vi "Chrg_Dschrg_new.vi"(0 "Data Task in":refnum<k21>, 1 "data task error in":errorcluster, 2 "#DAQ outputs (1-13)":i32, 3 "PS type":enum16{"NHR", "ITECH"}(ring), 4 "PS VISA in":refnum<visa-resource-name>, 5 "PS error in":errorcluster caption="NHR error in (no error)", 6 "DischargeCyclePath":path=path "C:/Users/ga11/Desktop/VI/results/3PtestCharge.lvm" caption="Filename", 7 "Battery Type":enum16{"30Q", "40T"}(ring), 8 "Charge/discharge":enum8{"Charge", "Discharge"}(ring), 9 "Charge/Discharge Voltage Setpoint":dbl format="%#.6g", 10 "CC or CCCV":enum16{"CC", "CCCV"}(ring), 11 "Current Setpoint":dbl format="%#.6g", 12 "Output Safety":T1, 13 "Current Cutoff":dbl) -> (14 "data task out":refnum<k21>, 15 "data task error out":errorcluster, 18 "PS VIS resource name out":refnum<visa-resource-name>, 19 "PS error out":errorcluster)   [LabVIEW 2020]
uses:
  Drivers-Essentials/NH Research Regenerative Test Series.lvlib
  Drivers-IT-M3400/IT-M3400.lvlib
  Drivers-Essentials/Read (Ave Current).vi
  Drivers-NHR-9200/NHR/Public/Data/Low Level/Fetch (Ave Voltage).vi
  <instrlib>/NH Research Regenerative Test Series/Public/Configure/Output Safety.ctl
panel:
  out "Read Ave Current (A)":dbl
  out "Read Ave Voltage (V)":dbl
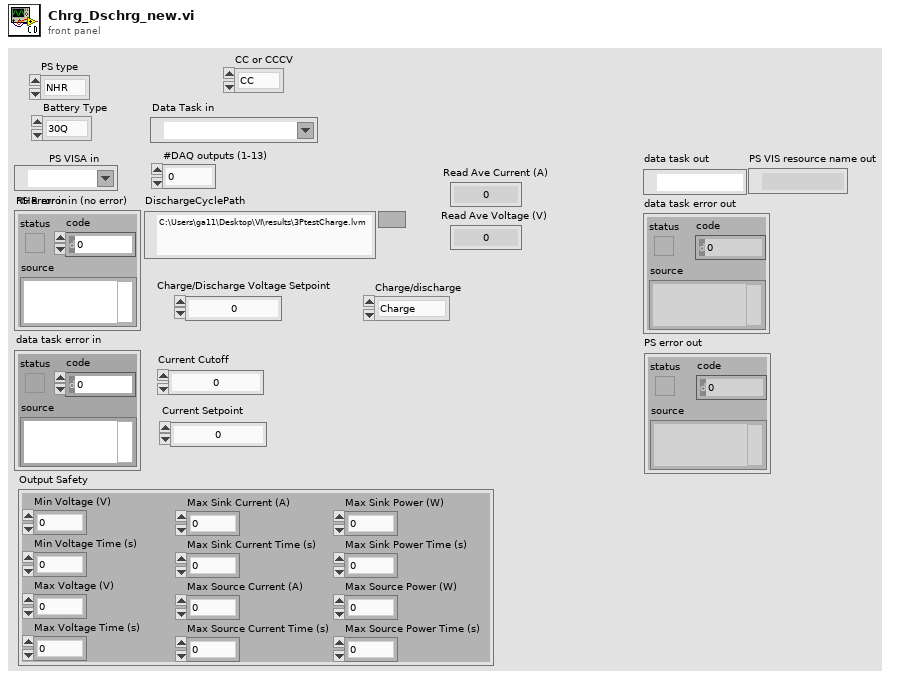
[diagram p1: front panel]
types:
  T1 = typedef "NH Research Regenerative Test Series.lvlib/Output Safety.ctl" = cluster{"Min Voltage (V)":dbl, "Min Voltage Time (s)":dbl, "Max Voltage (V)":dbl, "Max Voltage Time (s)":dbl, "Max Sink Current (A)":dbl, "Max Sink Current Time (s)":dbl, "Max Source Current (A)":dbl, "Max Source Current Time (s)":dbl, "Max Sink Power (W)":dbl, "Max Sink Power Time (s)":dbl, "Max Source Power (W)":dbl, "Max Source Power Time (s)":dbl}
  T2 = cluster{"Voltage Enabled":bool, "Current Enabled":bool, "Power Enabled":bool, "Resistance Enabled":bool}
  T3 = cluster{"Baud Rate":u32, "Parity":u16, "Data Bits":u16, "Stop Bits":u16, "Flow Control":u16}
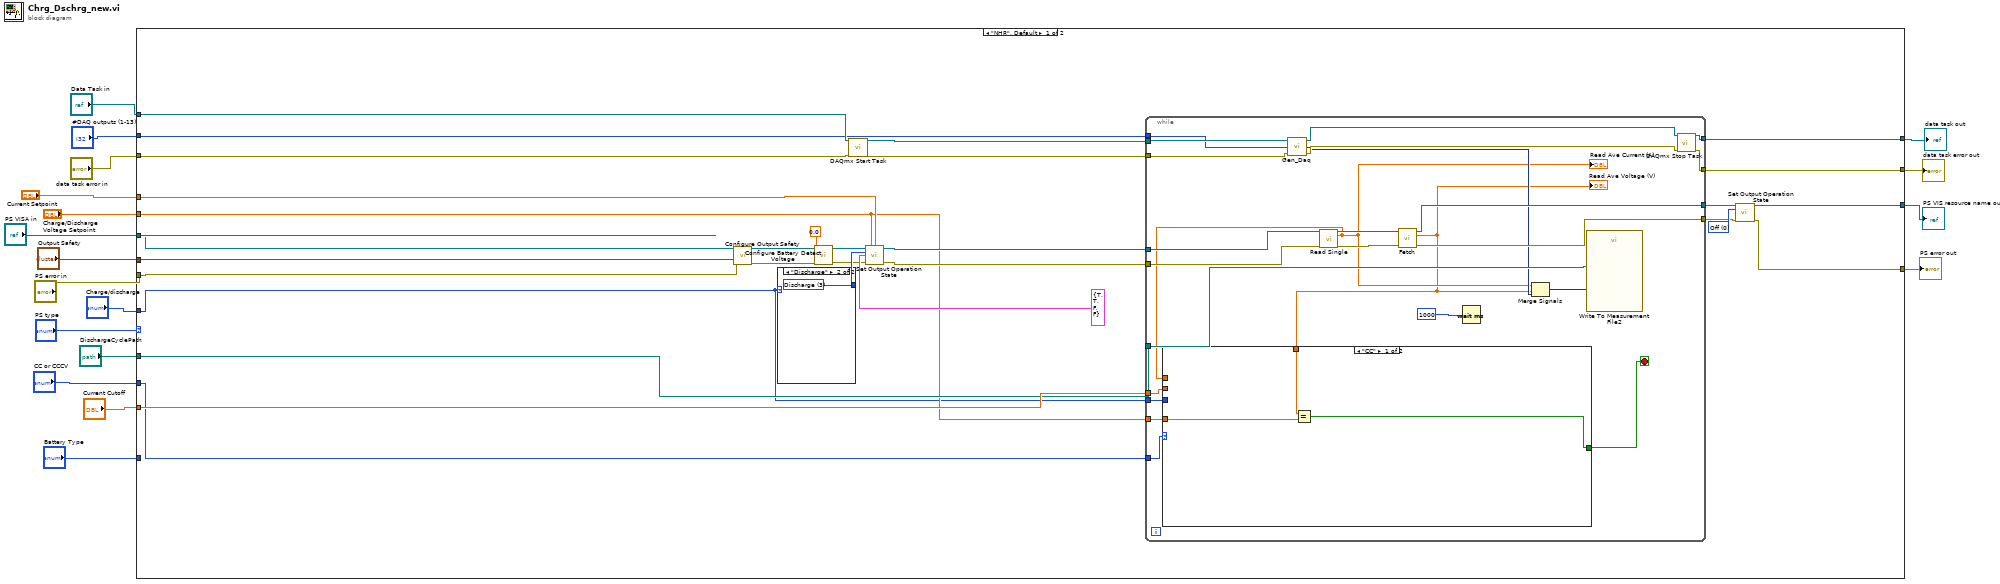
[diagram p0: block diagram]
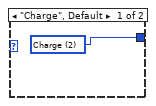
[diagram p2: hidden frame]
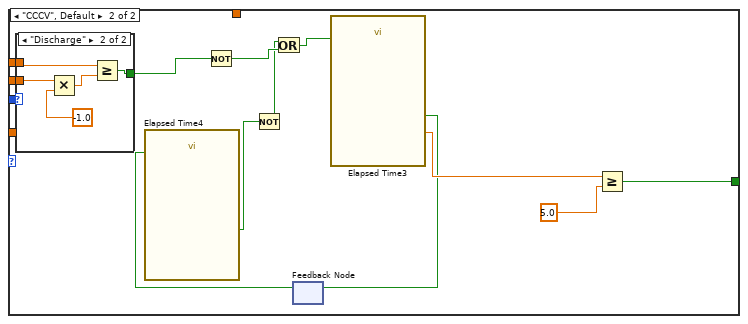
[diagram p3: hidden frame]
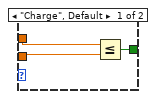
[diagram p4: hidden frame]
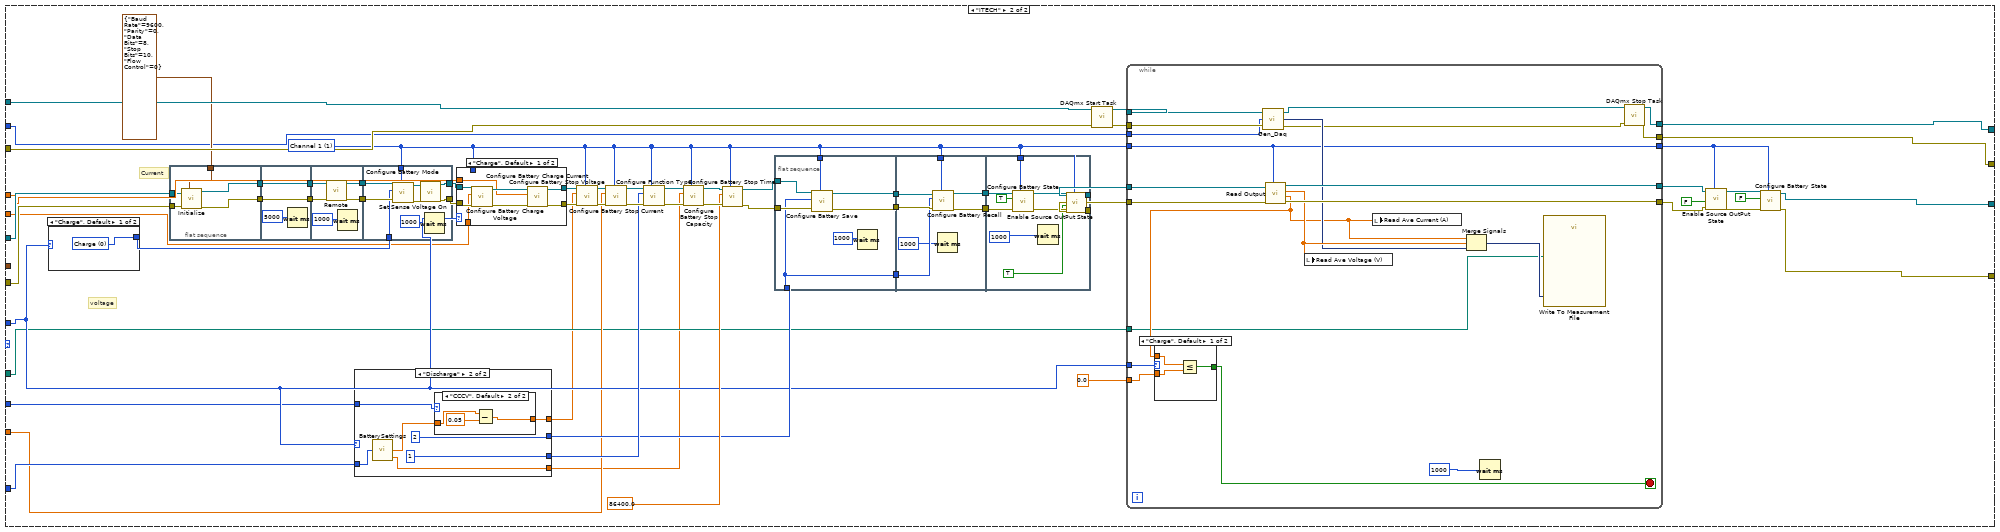
[diagram p5: hidden frame]
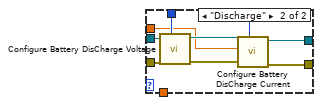
[diagram p6: hidden frame]
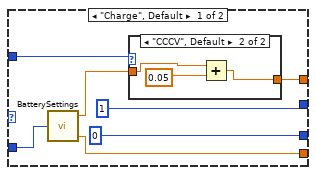
[diagram p7: hidden frame]
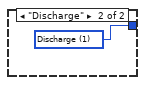
[diagram p10: hidden frame]
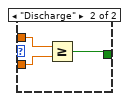
[diagram p11: hidden frame]
diagram:
  n1 = case shown="\"NHR\", Default" "PS type" {
    tunnel: "Charge/Discharge Voltage Setpoint" -> [w25 w104]
    tunnel: "Current Setpoint" -> [w27 w105]
    tunnel: "Current Cutoff" -> [w46 w109]
    tunnel: "DischargeCyclePath" -> [w43 w108]
    tunnel: "Data Task in" -> [w40 w150]
    tunnel: "data task error in" -> [w39 w151]
    tunnel: "PS VISA in" -> [w20 w107]
    tunnel: "PS error in" -> [w21 w106]
    tunnel: [w34 w149] -> w10
    tunnel: [w33 w147] -> w9
    tunnel: [w32 w148] -> w8
    tunnel: [w31 w146] -> w7
    tunnel: "#DAQ outputs (1-13)" -> [w28 w113]
    tunnel: "Battery Type" -> [_ w110]
    tunnel: "Charge/discharge" -> [w24 w111]
    tunnel: "CC or CCCV" -> [w26 w103]
    tunnel: "Output Safety" -> [w19 _]
    frame "NHR", Default {
      w38 = 0 items=["Off", "Standby", "Charge", "Discharge", "Battery"] ("Mode (0: Off)")
      n2 = call <instrlib>:"Configure Output Safety.vi"("VISA resource name"=w20, "Output Safety"=w19, "error in (no error)"=w21) -> ("VISA resource name out"=w23:refnum<visa-resource-name>, "error out"=w22:errorcluster)  [unwired: 11 in]
      n3 = case shown="\"Discharge\"" w24 {
        tunnel: [w49 w50] -> w44
        frame "Charge", Default {
          w49 = 2 items=["Off", "Standby", "Charge", "Discharge", "Battery"] ("Mode (0: Off)")
        }
        frame "Discharge" {
          w50 = 3 items=["Off", "Standby", "Charge", "Discharge", "Battery"] ("Mode (0: Off)")
        }
      }
      n4 = call "Configure Battery Detect Voltage.vi"("VISA resource name"=w23, "Battery Detect Voltage (0V)"=0.0, "error in (no error)"=w22) -> ("VISA resource name out"=w37:refnum<visa-resource-name>, "error out"=w36:errorcluster)  [unwired: 11 in]
      n5 = call <vilib>:"DAQmx Start Task.vi"("task/channels in"=w40, "error in"=w39) -> ("task out"=w42:refnum<k21>, "error out"=w41:errorcluster)  [unwired: 12 in]
      n6 = call "Set Output Operation State.vi"("VISA resource name"=w37, "Voltage Setpoint (0 V)"=w25, "Current Setpoint (0 A)"=w27, "Mode (0: Off)"=w44, "Enable"=T2 {"Voltage Enabled"=TRUE, "Current Enabled"=TRUE, "Power Enabled"=FALSE, "Resistance Enabled"=FALSE}, "error in (no error)"=w36) -> ("VISA resource name out"=w48:refnum<visa-resource-name>, "error out"=w47:errorcluster)  [unwired: 8 in]
      n7 = while {
        tunnel: w48 -> [w72]
        tunnel: w47 -> [w71]
        tunnel: w46 -> [w56]
        tunnel: w41 -> [w61]
        tunnel: w42 -> [w62]
        tunnel: w43 -> [w67]
        tunnel: [w66] -> w34
        tunnel: [w65] -> w32
        tunnel: [w64] -> w30
        tunnel: [w63] -> w29
        tunnel: w28 -> [w60]
        tunnel: w26 -> [w54]
        tunnel: w25 -> [w52]
        tunnel: w24 -> [w51]
        stop <- w68 stop-if-true
        n8 = call "Gen_Daq.vi"("error in"=w61, "#DAQ outputs (1-13)"=w60, "task/channels in"=w62) -> ("error out"=w58:errorcluster, "DaQ_output"=w57:dynamicdata, "task out"=w59:refnum<k21>)
        n9 = call-poly "Read Single.vi"("VISA resource name"=w72, "error in (no error)"=w71) -> ("VISA resource name out"=w73:refnum<visa-resource-name>, "Ave Current (A)"=w55:dbl, "error out"=w74:errorcluster)  [unwired: 11 in]
        "Read Ave Current (A)" <- w55
        n10 = call-poly "Fetch.vi"("VISA resource name"=w73, "error in (no error)"=w74) -> ("VISA resource name out"=w64:refnum<visa-resource-name>, "Ave Voltage (V)"=w53:dbl, "error out"=w63:errorcluster)  [unwired: 11 in]
        "Read Ave Voltage (V)" <- w53
        n11 = case shown="\"CC\"" w54 {
          tunnel: [w75 w84] -> w68
          tunnel: w56 -> [_ w81]
          tunnel: w55 -> [_ w80]
          tunnel: w53 -> [w77 _]
          tunnel: w52 -> [w76 _]
          tunnel: w51 -> [_ w78]
          frame "CC" {
            n12 = Equal?(x=w77, y=w76) -> (x = y?=w75:bool)
          }
          frame "CCCV", Default {
            n13 = case shown="\"Discharge\"" w78 {
              tunnel: w81 -> [w92 w97]
              tunnel: w80 -> [w93 w95]
              tunnel: [w91 w94] -> w79
              frame "Charge", Default {
                n14 = Less Or Equal?(x=w93, y=w92) -> (x <= y?=w91:bool)
              }
              frame "Discharge" {
                n15 = Multiply(x=w97, y=-1.0) -> (x*y=w96:dbl)
                n16 = Greater Or Equal?(x=w95, y=w96) -> (x >= y?=w94:bool)
              }
            }
            n17 = Not(x=w79) -> (.not. x?=w90:bool)
            n18 = feedback #1() -> (w82:bool)  [unwired: 1 in]
            n19 = call "Elapsed Time4"("Reset"=w82) -> ("Time has Elapsed"=w89:bool)  [unwired: 11 in, 7 out]
            n20 = Not(x=w89) -> (.not. x?=w88:bool)
            n21 = Or(x=w88, y=w90) -> (x .or. y?=w87:bool)
            n22 = call "Elapsed Time3"("Reset"=w87) -> ("Elapsed Time (s)"=w86:dbl, "Time has Elapsed"=w83:bool)  [unwired: 11 in, 6 out]
            n23 = feedback-in #1(w83) -> ()
            n24 = Greater Or Equal?(x=w86, y=5.0) -> (x >= y?=w84:bool)
          }
        }
        n25 = Wait (ms)(milliseconds to wait=1000) -> ()  [unwired: 1 out]
        n26 = Merge Signals "Merge Signals"(w55, w53, w57) -> (w70:dynamicdata)
        n27 = call "Write To Measurement File2"("Signals"=w70, "Filename"=w67) -> ()  [unwired: 15 in, 3 out]
        n28 = call <vilib>:"DAQmx Stop Task.vi"("task/channels in"=w59, "error in"=w58) -> ("task out"=w66:refnum<k21>, "error out"=w65:errorcluster)  [unwired: 12 in]
      }
      n29 = call "Set Output Operation State.vi"("VISA resource name"=w30, "Mode (0: Off)"=w38, "error in (no error)"=w29) -> ("VISA resource name out"=w33:refnum<visa-resource-name>, "error out"=w31:errorcluster)  [unwired: 11 in]
    }
    frame "ITECH" {
      w114 = 1 items=["Channel 1"=1, "Channel 2"=2, "Channel 3"=3, "Channel 4"=4, "Channel 5"=5, "Channel 6"=6, "Channel 7"=7, "Channel 8"=8, "Channel 8"=9, "Channel 10"=10, "Channel 11"=11, "Channel 12"=12, "Channel 13"=13, "Channel 14"=14, "Channel 15"=15, "Channel 16"=16] ("Channel")
      # "voltage"
      # "Current"
      n30 = case shown="\"Charge\", Default" w111 {
        tunnel: [w244 w245] -> w124
        frame "Charge", Default {
          w244 = u8 0 items=["Charge", "Discharge"] ("Battery Mode")
        }
        frame "Discharge" {
          w245 = u8 1 items=["Charge", "Discharge"] ("Battery Mode")
        }
      }
      n31 = flat-sequence {
        tunnel: [w160] -> w139
        tunnel: [w161] -> w138
        tunnel: T3 {"Baud Rate"=9600, "Parity"=0, "Data Bits"=8, "Stop Bits"=10, "Flow Control"=0} ("Serial Configuration") -> [w164]
        tunnel: w106 -> [w163]
        tunnel: w107 -> [w162]
        tunnel: w139 -> [w167]
        tunnel: [w167] -> w137
        tunnel: w138 -> [w166]
        tunnel: [w166] -> w136
        tunnel: [w172] -> w135
        tunnel: [w171] -> w134
        tunnel: w137 -> [w170]
        tunnel: w136 -> [w169]
        tunnel: w135 -> [w178]
        tunnel: w134 -> [w180]
        tunnel: w114 -> [w181]
        tunnel: w124 -> [w179]
        tunnel: [w174] -> w100
        tunnel: [w173] -> w99
        frame #0 {
          n32 = call "Initialize.vi"("Serial Configuration"=w164, "error in"=w163, "VISA resource name"=w162) -> ("error out"=w161:errorcluster, "VISA resource name out"=w160:refnum<visa-resource-name>)  [unwired: 7 in]
        }
        frame #1 {
          n33 = Wait (ms)(milliseconds to wait=5000) -> ()  [unwired: 1 out]
        }
        frame #2 {
          n34 = call "Remote.vi"("error in"=w169, "VISA resource name"=w170) -> ("error out"=w171:errorcluster, "VISA resource name out"=w172:refnum<visa-resource-name>)  [unwired: 8 in]
          n35 = Wait (ms)(milliseconds to wait=1000) -> ()  [unwired: 1 out]
        }
        frame #3 {
          n36 = call "Configure Battery Mode.vi"("Channel"=w181, "error in"=w180, "Battery Mode"=w179, "VISA resource name"=w178) -> ("error out"=w175:errorcluster, "VISA resource name out"=w176:refnum<visa-resource-name>)  [unwired: 6 in]
          n37 = call "Set Sense Voltage On.vi"("error in"=w175, "VISA resource name"=w176) -> ("error out"=w174:errorcluster, "VISA resource name out"=w173:refnum<visa-resource-name>)  [unwired: 8 in]
          n38 = Wait (ms)(milliseconds to wait=1000) -> ()  [unwired: 1 out]
        }
      }
      n39 = case shown="\"Discharge\"" w111 {
        tunnel: w110 -> [w228 w233]
        tunnel: [u8 0 ("File") u8 1 ("File")] -> w118
        tunnel: [u8 1 ("File") u8 2 ("File")] -> w117
        tunnel: [w225 w237] -> w101
        tunnel: w103 -> [w222 w236]
        tunnel: [w223 w235] -> w102
        frame "Charge", Default {
          n40 = call "BatterySettings.vi"("Battery Type"=w228) -> ("RatedCapacity (Ah)"=w225:dbl, "Max Voltage (V)"=w224:dbl)  [unwired: 2 in, 1 out]
          n41 = case shown="\"CCCV\", Default" w222 {
            tunnel: w224 -> [w229 w231]
            tunnel: [w229 w230] -> w223
            frame "CC" {
            }
            frame "CCCV", Default {
              n42 = Add(x=w231, y=0.05) -> (x+y=w230:dbl)
            }
          }
        }
        frame "Discharge" {
          n43 = call "BatterySettings.vi"("Battery Type"=w233) -> ("RatedCapacity (Ah)"=w237:dbl, "Min Voltage (V)"=w234:dbl)  [unwired: 2 in, 1 out]
          n44 = case shown="\"CCCV\", Default" w236 {
            tunnel: w234 -> [w240 w242]
            tunnel: [w240 w241] -> w235
            frame "CC" {
            }
            frame "CCCV", Default {
              n45 = Subtract(x=w242, y=0.05) -> (x-y=w241:dbl)
            }
          }
        }
      }
      n46 = case shown="\"Charge\", Default" w111 {
        tunnel: w99 -> [w206 w221]
        tunnel: w100 -> [w213 w220]
        tunnel: [w209 w217] -> w129
        tunnel: [w208 w216] -> w128
        tunnel: w114 -> [_ w215]
        tunnel: w105 -> [w210 w214]
        tunnel: w104 -> [w207 _]
        frame "Charge", Default {
          n47 = call "Configure Battery Charge Voltage.vi"("error in"=w213, "Charge Voltage(V)"=w207, "VISA resource name"=w206) -> ("error out"=w211:errorcluster, "VISA resource name out"=w212:refnum<visa-resource-name>)  [unwired: 6 in]
          n48 = call "Configure Battery Charge Current.vi"("error in"=w211, "Charge Current(A)"=w210, "VISA resource name"=w212) -> ("error out"=w208:errorcluster, "VISA resource name out"=w209:refnum<visa-resource-name>)  [unwired: 7 in]
        }
        frame "Discharge" {
          n49 = call "Configure Battery DisCharge Voltage.vi"("Channel"=w215, "error in"=w220, "VISA resource name"=w221) -> ("error out"=w218:errorcluster, "VISA resource name out"=w219:refnum<visa-resource-name>)  [unwired: 7 in]
          n50 = call "Configure Battery DisCharge Current.vi"("Channel"=w215, "error in"=w218, "Discharge Current(A)"=w214, "VISA resource name"=w219) -> ("error out"=w216:errorcluster, "VISA resource name out"=w217:refnum<visa-resource-name>)  [unwired: 6 in]
        }
      }
      n51 = call "Configure Battery Stop Voltage.vi"("Channel"=w114, "error in"=w128, "Stop Voltage(V)"=w102, "VISA resource name"=w129) -> ("error out"=w132:errorcluster, "VISA resource name out"=w133:refnum<visa-resource-name>)  [unwired: 6 in]
      n52 = call "Configure Battery Stop Current.vi"("Channel"=w114, "error in"=w132, "Stop Current(A)"=w109, "VISA resource name"=w133) -> ("error out"=w120:errorcluster, "VISA resource name out"=w122:refnum<visa-resource-name>)  [unwired: 6 in]
      n53 = call "Configure Function Type.vi"("Channel"=w114, "error in"=w120, "Function Type"=w118, "VISA resource name"=w122) -> ("error out"=w119:errorcluster, "VISA resource name out"=w121:refnum<visa-resource-name>)  [unwired: 6 in]
      n54 = call "Configure Battery Stop Capacity.vi"("Channel"=w114, "error in"=w119, "Stop Capacity(Ah)"=w101, "VISA resource name"=w121) -> ("error out"=w130:errorcluster, "VISA resource name out"=w131:refnum<visa-resource-name>)  [unwired: 6 in]
      n55 = call "Configure Battery Stop Time.vi"("Channel"=w114, "error in"=w130, "Stop Time(S)"=86400.0, "VISA resource name"=w131) -> ("error out"=w126:errorcluster, "VISA resource name out"=w125:refnum<visa-resource-name>)  [unwired: 6 in]
      n56 = flat-sequence {
        tunnel: w117 -> [w187]
        tunnel: w114 -> [w182]
        tunnel: [w185] -> w144
        tunnel: [w187] -> w143
        tunnel: [w184] -> w142
        tunnel: w126 -> [w188]
        tunnel: w125 -> [w186]
        tunnel: [w191] -> w141
        tunnel: [w192] -> w140
        tunnel: w144 -> [w195]
        tunnel: w143 -> [w194]
        tunnel: w142 -> [w193]
        tunnel: w114 -> [w189]
        tunnel: [w199] -> w116
        tunnel: [w198] -> w115
        tunnel: w114 -> [w197]
        tunnel: w141 -> [w205]
        tunnel: w140 -> [w204]
        frame #0 {
          n57 = call "Configure Battery Save.vi"("Channel"=w182, "error in"=w188, "File"=w187, "VISA resource name"=w186) -> ("error out"=w185:errorcluster, "VISA resource name out"=w184:refnum<visa-resource-name>)  [unwired: 6 in]
          n58 = Wait (ms)(milliseconds to wait=1000) -> ()  [unwired: 1 out]
        }
        frame #1 {
          n59 = call "Configure Battery Recall.vi"("Channel"=w189, "error in"=w195, "File"=w194, "VISA resource name"=w193) -> ("error out"=w192:errorcluster, "VISA resource name out"=w191:refnum<visa-resource-name>)  [unwired: 6 in]
          n60 = Wait (ms)(milliseconds to wait=1000) -> ()  [unwired: 1 out]
        }
        frame #2 {
          n61 = call "Configure Battery State.vi"("Channel"=w197, "error in"=w204, "State"=TRUE, "VISA resource name"=w205) -> ("error out"=w202:errorcluster, "VISA resource name out"=w203:refnum<visa-resource-name>)  [unwired: 6 in]
          n62 = Wait (ms)(milliseconds to wait=1000) -> ()  [unwired: 1 out]
          n63 = call "Enable Source OutPut State.vi"("Channel"=w197, "error in"=w202, "State"=TRUE ("Enable Output|Intput"), "VISA resource name"=w203) -> ("error out"=w198:errorcluster, "VISA resource name out"=w199:refnum<visa-resource-name>)  [unwired: 6 in]
        }
      }
      n64 = call <vilib>:"DAQmx Start Task.vi"("task/channels in"=w150, "error in"=w151) -> ("task out"=w153:refnum<k21>, "error out"=w152:errorcluster)  [unwired: 12 in]
      n65 = while {
        tunnel: [w266] -> w155
        tunnel: [w265] -> w154
        tunnel: w153 -> [w262]
        tunnel: w152 -> [w261]
        tunnel: [w258] -> w149
        tunnel: [w257] -> w148
        tunnel: 0.0 -> [w254]
        tunnel: w116 -> [w251]
        tunnel: w115 -> [w250]
        tunnel: w114 -> [w248]
        tunnel: w113 -> [w249]
        tunnel: [w248] -> w112
        tunnel: w111 -> [w247]
        tunnel: w108 -> [w246]
        stop <- w252 stop-if-true
        n66 = call "Gen_Daq.vi"("error in"=w261, "#DAQ outputs (1-13)"=w249, "task/channels in"=w262) -> ("error out"=w259:errorcluster, "DaQ_output"=w263:dynamicdata, "task out"=w260:refnum<k21>)
        n67 = call "Read Output.vi"("Channel"=w248, "error in"=w250, "VISA resource name"=w251) -> ("error out"=w265:errorcluster, "Read Current(A)"=w253:dbl, "Read Voltage(V)"=w264:dbl, "VISA resource name out"=w266:refnum<visa-resource-name>)  [unwired: 5 in]
        n68 = case shown="\"Charge\", Default" w247 {
          tunnel: w254 -> [w268 w271]
          tunnel: w253 -> [w269 w272]
          tunnel: [w267 w270] -> w252
          frame "Charge", Default {
            n69 = Less Or Equal?(x=w269, y=w268) -> (x <= y?=w267:bool)
          }
          frame "Discharge" {
            n70 = Greater Or Equal?(x=w272, y=w271) -> (x >= y?=w270:bool)
          }
        }
        n71 = local write "Read Ave Voltage (V)"(w264) -> ()
        n72 = local write "Read Ave Current (A)"(w253) -> ()
        n73 = Merge Signals "Merge Signals"(w253, w264, w263) -> (w256:dynamicdata)
        n74 = Wait (ms)(milliseconds to wait=1000) -> ()  [unwired: 1 out]
        n75 = call "Write To Measurement File"("Signals"=w256, "Filename"=w246) -> ()  [unwired: 15 in, 3 out]
        n76 = call <vilib>:"DAQmx Stop Task.vi"("task/channels in"=w260, "error in"=w259) -> ("task out"=w258:refnum<k21>, "error out"=w257:errorcluster)  [unwired: 12 in]
      }
      n77 = call "Enable Source OutPut State.vi"("Channel"=w112, "error in"=w154, "State"=FALSE, "VISA resource name"=w155) -> ("error out"=w158:errorcluster, "VISA resource name out"=w159:refnum<visa-resource-name>)  [unwired: 6 in]
      n78 = call "Configure Battery State.vi"("Channel"=w112, "error in"=w158, "State"=FALSE, "VISA resource name"=w159) -> ("error out"=w146:errorcluster, "VISA resource name out"=w147:refnum<visa-resource-name>)  [unwired: 6 in]
    }
  }
  "data task out" <- w10
  "PS VIS resource name out" <- w9
  "data task error out" <- w8
  "PS error out" <- w7
